vi "_PC_Pub_Var2String.vi"(1 "Array of VData":variant[](array[variant]), 2 "Output Type":T1[](array[typedef]) format="%.0x") -> (0 "String Array":string[](array[string]))   [LabVIEW 2018]
uses:
  <userlib>/_OpenG.lib/lvdata/lvdata.llb/Type Descriptor Enumeration__ogtk.ctl
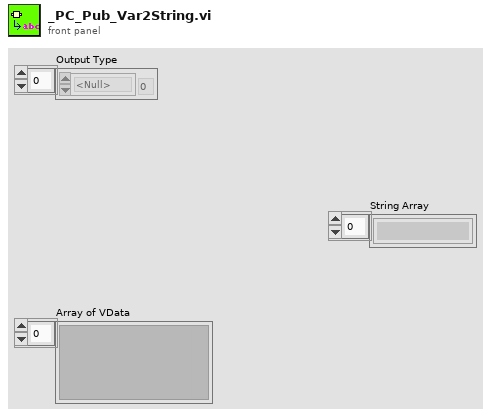
[diagram p1: front panel]
types:
  T1 = typedef "Type Descriptor Enumeration__ogtk.ctl" = enum8{"<Null>", "I8", "I16", "I32", "I64", "U8", "U16", "U32", "U64", "SGL", "DBL", "EXT", "CSG", "CDB", "CXT", "0x0F", "0x10", "0x11", "0x12", "0x13", "0x14", "Enum U8", "Enum U16", "Enum U32", "Enum U64", "SGL PQ", "DBL PQ", "EXT PQ", "CSG PQ", "CDB PQ", "CXT PQ", "0x1F", "0x20", "Boolean", "0x22", "0x23", "0x24", "0x25", "0x26", "0x27", "0x28", "0x29", "0x2A", "0x2B", "0x2C", "0x2D", "0x2E", "0x2F", "String", "0x31", "Path", "Pict", "0x34", "0x35", "0x36", "DAQ", "0x38", "0x39", "0x3A", "0x3B", "0x3C", "0x3D", "0x3E", "0x3F", "Array", "0x41", "0x42", "0x43", "0x44", "0x45", "0x46", "0x47", "0x48", "0x49", "0x4A", "0x4B", "0x4C", "0x4D", "0x4E", "0x4F", "Cluster", "0x51", "0x52", "Variant", "Waveform", "0x55", "0x56", "0x57", "0x58", "0x59", "0x5A", "0x5B", "0x5C", "0x5D", "0x5E", "0x5F", "0x60", "0x61", "0x62", "0x63", "0x64", "0x65", "0x66", "0x67", "0x68", "0x69", "0x6A", "0x6B", "0x6C", "0x6D", "0x6E", "0x6F", "Refnum"}
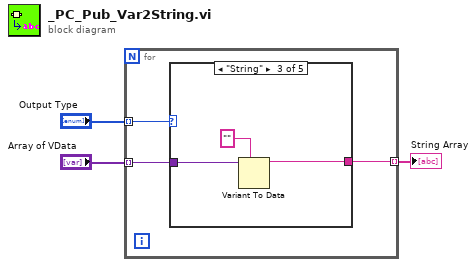
[diagram p0: block diagram]
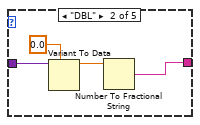
[diagram p3: hidden frame]
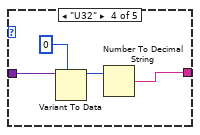
[diagram p4: hidden frame]
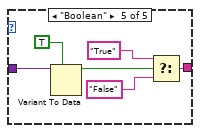
[diagram p5: hidden frame]
diagram:
  n1 = for {
    tunnel: "Output Type" -> [w6] mode=indexing
    tunnel: "Array of VData" -> [w5] mode=indexing
    tunnel: [w4] -> w1 mode=indexing
    n2 = case shown="\"String\"" w6 {
      tunnel: w5 -> [_ w10 w13 w17 w23]
      tunnel: [_ w7 w11 w14 w20] -> w4
      frame "<Null>", Default {
      }
      frame "DBL" {
        n3 = Variant To Data(type=0.0, Variant=w10) -> (data=w8:dbl)  [unwired: 1 in, 1 out]
        n4 = Number To Fractional String(number=w8) -> (F-format string=w7:string)  [unwired: 3 in]
      }
      frame "String" {
        n5 = Variant To Data(type="", Variant=w13) -> (data=w11:string)  [unwired: 1 in, 1 out]
      }
      frame "U32" {
        n6 = Variant To Data(type=u32 0, Variant=w17) -> (data=w15:u32)  [unwired: 1 in, 1 out]
        n7 = Number To Decimal String(number=w15) -> (decimal integer string=w14:string)  [unwired: 1 in]
      }
      frame "Boolean" {
        n8 = Variant To Data(type=TRUE, Variant=w23) -> (data=w21:bool)  [unwired: 1 in, 1 out]
        n9 = Select(t="True", s=w21, f="False") -> (s? t:f=w20:string)
      }
    }
  }
  "String Array" <- w1
